vi "WriteBufferLocation.vi"(8 "error in (no error)":errorcluster, 10 "block params":T1, 11 "map in":T3) -> (0 "error out":errorcluster, 3 "map out":T3)   [LabVIEW 2017, in "DVRBuffer.lvlib"]
uses:
  <vilib>/addons/InsightCM/Devices/Shared/Common/DVRBuffer/DVRBuffer.lvlib
  <vilib>/addons/PointValueMap/controls/PointMap.ctl
  <vilib>/addons/InsightCM/Devices/Shared/Common/DataAccumulator/controls/BlockParams.ctl
  <vilib>/addons/InsightCM/Devices/Shared/Common/DVRBuffer/controls/BufferLocation.ctl
  <vilib>/addons/PointValueMap/subVIs/Point_Write_variant.vi
  <vilib>/addons/PointValueMap/subVIs/Point_Write_double.vi
  <vilib>/addons/PointValueMap/PointValueMap.lvlib
  <vilib>/addons/InsightCM/Devices/Shared/Common/DataAccumulator/DataAccumulator.lvlib
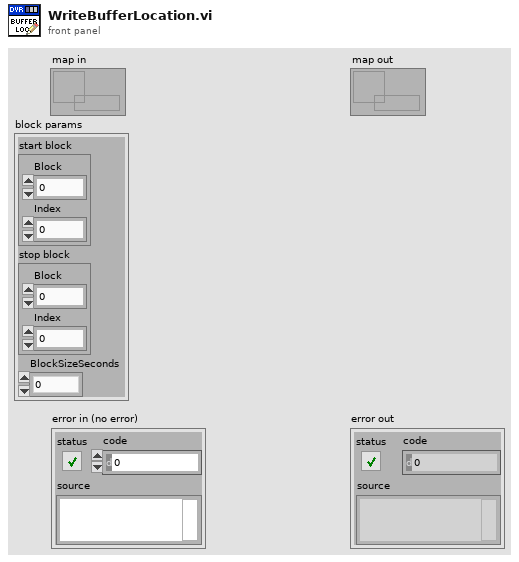
[diagram p1: front panel]
types:
  T1 = typedef "DataAccumulator.lvlib/BlockParams.ctl" = cluster{"start block":T2, "stop block":T2, "BlockSizeSeconds":dbl}
  T2 = typedef "DVRBuffer.lvlib/BufferLocation.ctl" = cluster{"Block":u32, "Index":i32}
  T3 = typedef "PointValueMap.lvlib/PointMap.ctl" = refnum<data-value>
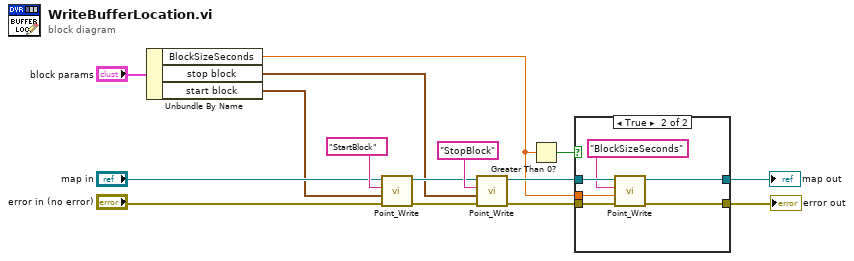
[diagram p0: block diagram]
diagram:
  n1 = Unbundle By Name("block params") -> ("BlockSizeSeconds"=w3:dbl, "stop block"=w8:T2, "start block"=w9:T2)
  n2 = call-poly <vilib>:"Point_Write.vi"("Error In"="error in (no error)", "Value"=w9, "Tag"="StartBlock", "Map"="map in") -> ("Error Out"=w10:errorcluster, "Map Out"=w11:T3)  [unwired: 6 in]
  n3 = call-poly <vilib>:"Point_Write.vi"("Error In"=w10, "Value"=w8, "Tag"="StopBlock", "Map"=w11) -> ("Error Out"=w6:errorcluster, "Map Out"=w7:T3)  [unwired: 6 in]
  n4 = Greater Than 0?(x=w3) -> (x > 0?=w2:bool)
  n5 = case shown="True" w2 {
    tunnel: w7 -> [w17 w23]
    tunnel: w6 -> [w16 w22]
    tunnel: [w16 w21] -> w5
    tunnel: [w17 w20] -> w4
    tunnel: w3 -> [_ w18]
    frame False {
    }
    frame True {
      n6 = call-poly <vilib>:"Point_Write.vi"("Error In"=w22, "Value"=w18, "Tag"="BlockSizeSeconds", "Map"=w23) -> ("Error Out"=w21:errorcluster, "Map Out"=w20:T3)  [unwired: 6 in]
    }
  }
  "error out" <- w5
  "map out" <- w4
